vi "Write Blue robots.vi"(8 "error in (no error)":errorcluster, 10 "Blue robots":refnum<class "Robot.lvclass">[](array[class]), 11 "Camera in":refnum<class "Camera.lvclass">) -> (0 "error out":errorcluster, 3 "Camera out":refnum<class "Camera.lvclass">)   [LabVIEW 2018, in "Camera.lvclass"]
uses:
  Camera.lvclass
  Robot_class/Robot.lvclass
  Camera.lvclass/Camera.ctl
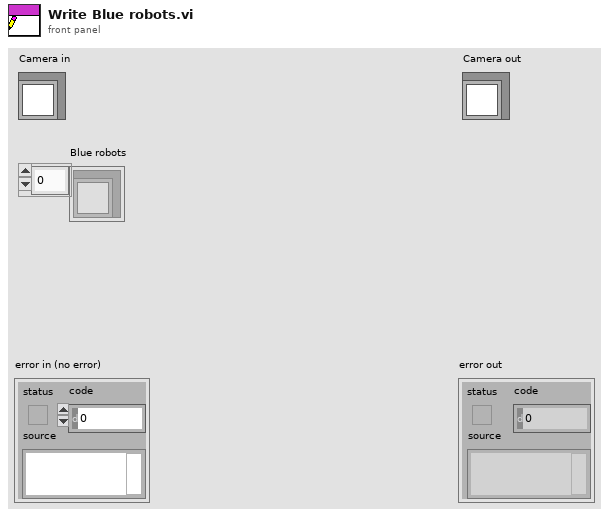
[diagram p1: front panel]
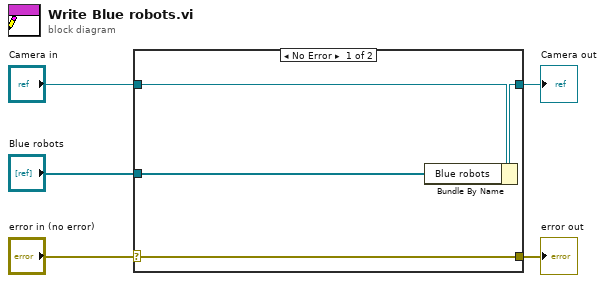
[diagram p0: block diagram]
diagram:
  n1 = case shown="No Error" "error in (no error)" {
    selector: "error in (no error)" -> [w9 w10]
    tunnel: [w9 w10] -> w4
    tunnel: [w7 w11] -> w2
    tunnel: "Camera in" -> [w8 w11]
    tunnel: "Blue robots" -> [w6 _]
    frame No Error {
      n2 = Bundle By Name(cluster=w8, "Blue robots"=w6) -> (w7:refnum<class "Camera.lvclass">)
    }
    frame Error {
    }
  }
  "error out" <- w4
  "Camera out" <- w2
